vi "Quit all tasks.vi"(4 "error in":errorcluster, 5 "Main cluster in":T1) -> (0 "error out":errorcluster, 1 "Main cluster out":T1)   [LabVIEW 2010]
uses:
  Main_cluster.ctl
  <vilib>/vision/Image Controls.llb/IMAQ Image.ctl
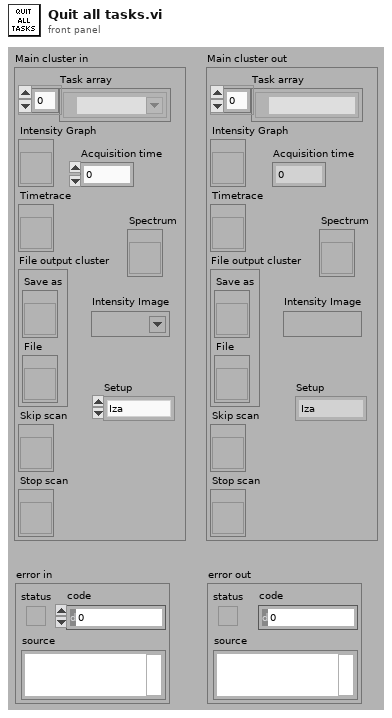
[diagram p1: front panel]
types:
  T1 = typedef "Main_cluster.ctl" = cluster{"Task array":refnum<k21>[], "Intensity Graph":refnum<vi>, "Timetrace":refnum<vi>, "File output cluster":cluster{"Save as":refnum<vi>, "File":refnum<vi>}, "Skip scan":refnum<vi>, "Stop scan":refnum<vi>, "Acquisition time":dbl, "Setup":enum16{"Iza", "Lukasz"}, "Spectrum":refnum<vi>, "Intensity Image":T2}
  T2 = typedef "IMAQ Image.ctl" = refnum<image>
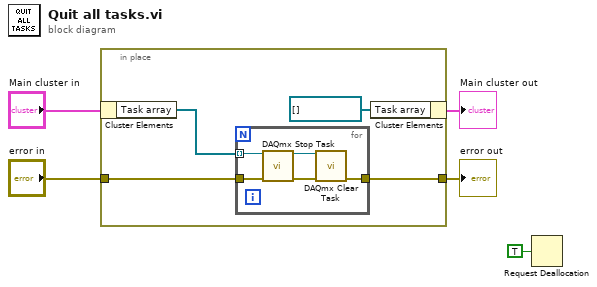
[diagram p0: block diagram]
diagram:
  n1 = in-place {
    in-place-border: [w9] -> w5
    in-place-border: "error in" -> [w8]
    n2 = in-place-cluster #1("Main cluster in") -> ("Task array"=w7:refnum<k21>[])
    n3 = for {
      tunnel: w8 -> [w12]
      tunnel: [w11] -> w9
      tunnel: w7 -> [w10] mode=indexing
      n4 = call <vilib>:"DAQmx Stop Task.vi"("task/channels in"=w10, "error in"=w12) -> ("task out"=w14:refnum<k21>, "error out"=w13:errorcluster)  [unwired: 12 in]
      n5 = call <vilib>:"DAQmx Clear Task.vi"("task in"=w14, "error in"=w13) -> ("error out"=w11:errorcluster)  [unwired: 13 in]
    }
    n6 = in-place-cluster #1("Task array"=refnum<k21>[] []) -> (→"Main cluster out":T1)
  }
  "error out" <- w5
  n7 = Request Deallocation(TRUE ("flag")) -> ()
